vi "编辑文本.vi"(8 "error in (no error)":errorcluster caption="错误输入（无错误）", 9 "扫描代码":i16, 11 "程序 输入":refnum<class "程序.lvclass">) -> (0 "error out":errorcluster caption="错误输出", 3 "程序 输出":refnum<class "程序.lvclass">)   [LabVIEW 2020, in "程序.lvclass"]
uses:
  D:/SuperPython-master/ScintillaNET.dll
  ScintillaNET.dll
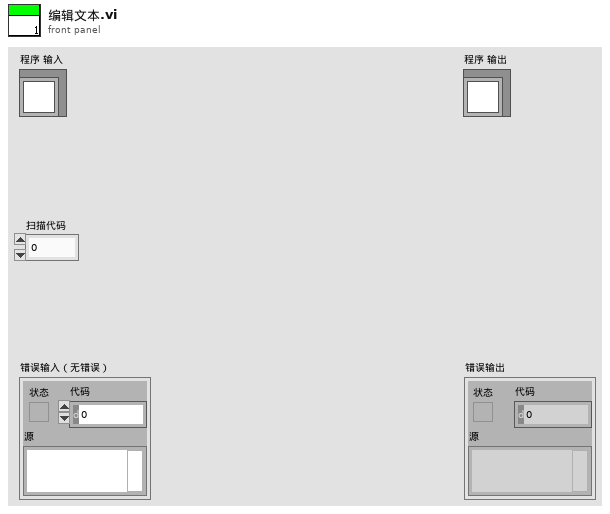
[diagram p1: front panel]
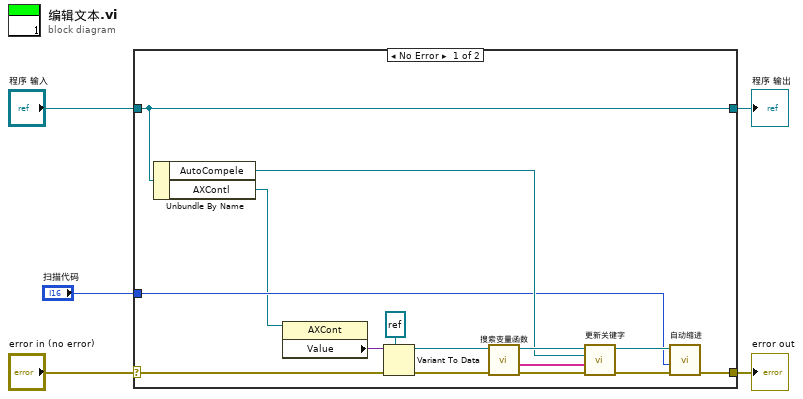
[diagram p0: block diagram]
diagram:
  n1 = case shown="No Error" "error in (no error)" {
    selector: "error in (no error)" -> [w7 w22]
    tunnel: [w12 w22] -> w4
    tunnel: [w15 w21] -> w2
    tunnel: "程序 输入" -> [w15 w21]
    tunnel: "扫描代码" -> [w13 _]
    frame No Error {
      n2 = Unbundle By Name(w15) -> ("AutoCompele"=w14:refnum<k24>, "AXContl"=w9:refnum<vi>)
      n3 = property class="AXCont"(reference=w9) -> ("Value"=w11:variant)  [unwired: 1 in, 2 out]
      n4 = Variant To Data(error in=w7, type=refnum<k24> refnum ("Scintilla"), Variant=w11) -> (data=w8:refnum<k24>, error out=w6:errorcluster)
      n5 = call "搜索变量函数.vi"("错误输入"=w6, "引用"=w8) -> ("错误输出"=w18:errorcluster, "输出数组"=w20:string[], "引用输出"=w19:refnum<k24>)  [unwired: 7 in]
      n6 = call "更新关键字.vi"("错误输入"=w18, "变量函数"=w20, "引用 2"=w14, "引用"=w19) -> ("错误输出"=w16:errorcluster, "引用输出"=w17:refnum<k24>)  [unwired: 5 in, 1 out]
      n7 = call "自动缩进.vi"("错误输入"=w16, "扫描代码"=w13, "引用"=w17) -> ("错误输出"=w12:errorcluster)  [unwired: 7 in, 1 out]
    }
    frame Error {
    }
  }
  "error out" <- w4
  "程序 输出" <- w2
